vi "set_ROI.vi"(11 "Cursor List":T1) -> (0 "Row End":dbl, 1 "RowStart":dbl, 2 "ColEnd":dbl, 3 "ColStart":dbl)   [LabVIEW 2016]
uses:
  <vilib>/Utility/miscctls.llb/LVCursorListTypeDef.ctl
panel:
  out "Intensity Graph":dbl[][](graph)
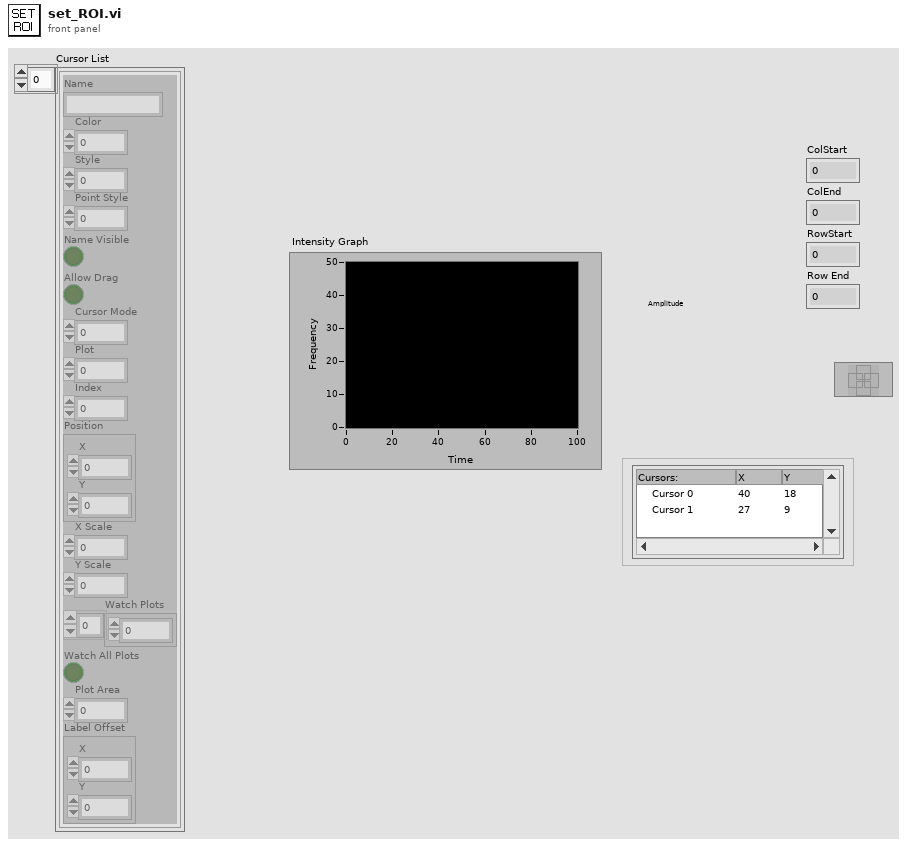
[diagram p1: front panel]
types:
  T1 = typedef "LVCursorListTypeDef.ctl" = cluster{"Name":string, "Color":u32, "Style":u8, "Point Style":u8, "Name Visible":bool, "Allow Drag":bool, "Cursor Mode":u32, "Plot":i32, "Index":i32, "Position":cluster{"X":dbl, "Y":dbl}, "X Scale":u32, "Y Scale":u32, "Watch Plots":i32[], "Watch All Plots":bool, "Plot Area":i32, "Label Offset":cluster{"X":dbl, "Y":dbl}}[]
  T2 = cluster{"Name":string, "Color":u32, "Style":u8, "Point Style":u8, "Name Visible":bool, "Allow Drag":bool, "Cursor Mode":u32, "Plot":i32, "Index":i32, "Position":cluster{"X":dbl, "Y":dbl}, "X Scale":u32, "Y Scale":u32, "Watch Plots":i32[], "Watch All Plots":bool, "Plot Area":i32, "Label Offset":cluster{"X":dbl, "Y":dbl}}
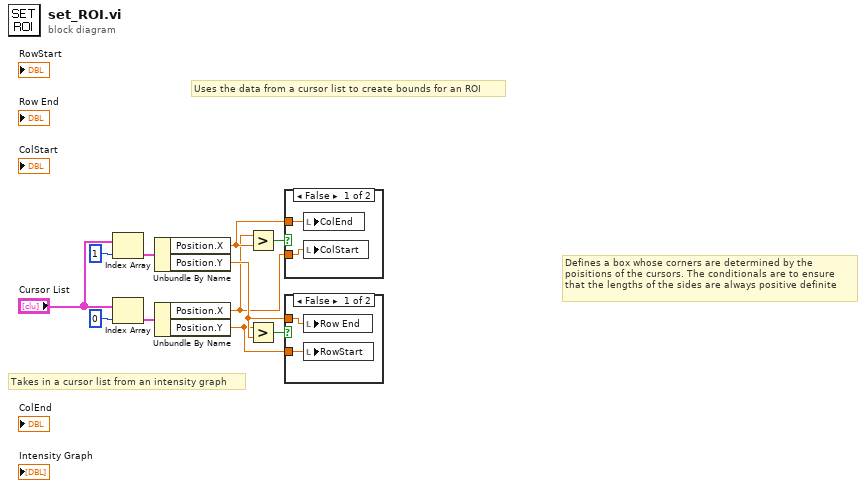
[diagram p0: block diagram]
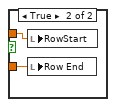
[diagram p2: hidden frame]
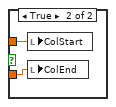
[diagram p3: hidden frame]
diagram:
  # "Defines a box whose corners are determined by the\npoisitions of the cursors. The conditionals are to ensure\nthat the lengths of the sides are always positive definite"
  # "Uses the data from a cursor list to create bounds for an ROI"
  # "Takes in a cursor list from an intensity graph"
  n1 = Index Array(array="Cursor List", index=1) -> (element=w7:T2)
  n2 = Index Array(array="Cursor List", index=0) -> (element=w8:T2)
  n3 = Unbundle By Name(w7) -> ("Position.X"=w2:dbl, "Position.Y"=w4:dbl)
  n4 = Unbundle By Name(w8) -> ("Position.X"=w1:dbl, "Position.Y"=w3:dbl)
  n5 = Greater?(x=w1, y=w2) -> (0:w5:bool)
  n6 = Greater?(x=w3, y=w4) -> (0:w6:bool)
  n7 = case shown="False" w5 {
    tunnel: w2 -> [w12 w15]
    tunnel: w1 -> [w13 w14]
    frame False {
      n8 = local write "ColEnd"(w12) -> ()
      n9 = local write "ColStart"(w13) -> ()
    }
    frame True {
      n10 = local write "ColStart"(w15) -> ()
      n11 = local write "ColEnd"(w14) -> ()
    }
  }
  n12 = case shown="False" w6 {
    tunnel: w4 -> [w17 w19]
    tunnel: w3 -> [w16 w18]
    frame False {
      n13 = local write "Row End"(w17) -> ()
      n14 = local write "RowStart"(w16) -> ()
    }
    frame True {
      n15 = local write "RowStart"(w19) -> ()
      n16 = local write "Row End"(w18) -> ()
    }
  }
